vi "UI Array to KH Settings.vi"(4 "Bandwidth Filter":bool, 6 "DC Coupled":bool, 7 "KH Ch Ring":refnum<vi>, 8 "Default Shunt Resistor":T1=enum."50 Ohms", 9 "KH All Buttons":T15(ring), 10 "UI Channels []":T2[](array[typedef]) {"KH"."Channel" items=["A 1"]}, 11 "KH Ch Settings in":cluster{"Channel Setting":T10}[](array[cluster])) -> (2 "UI Channels [] out":T2[](array[typedef]) {"KH"."Channel" items=["A 1"]}, 3 "KH Ch Settings out":cluster{"Channel Setting":T10}[](array[cluster]))   [LabVIEW 2016, in "Control Experiment UI.lvclass"]
uses:
  Control Experiment UI.lvclass
  Typedefs/UI Channels--Cluster.ctl
  Typedefs/UI Channels.AI--Cluster.ctl
  Typedefs/UI Channels.Device--Cluster.ctl
  Control Experiment SM/Typedefs/KH Mode-enum.ctl
  Typedefs/UI Channels.KH--Cluster.ctl
  <userlib>/LevyLab/Krohn Hite 7008/typedefs/Input Configuration-Enum.ctl
  <userlib>/LevyLab/Krohn Hite 7008/typedefs/Gain-Enum.ctl
  <userlib>/LevyLab/Krohn Hite 7008/typedefs/Shunt-Enum.ctl
  Typedefs/UI Channels.AO--Cluster.ctl
  <userlib>/LevyLab/Krohn Hite 7008/typedefs/SetAll-Array.ctl
  <userlib>/LevyLab/Krohn Hite 7008/typedefs/SetAll-Cluster.ctl
  <userlib>/LevyLab/Krohn Hite 7008/typedefs/Channel-Enum.ctl
  <userlib>/LevyLab/Krohn Hite 7008/typedefs/Filter-Enum.ctl
  <userlib>/LevyLab/Krohn Hite 7008/typedefs/Coupling-Enum.ctl
  <userlib>/LevyLab/Krohn Hite 7008/Instrument.KH7008.lvclass
  Control Experiment SM/Control Experiment SM.lvclass
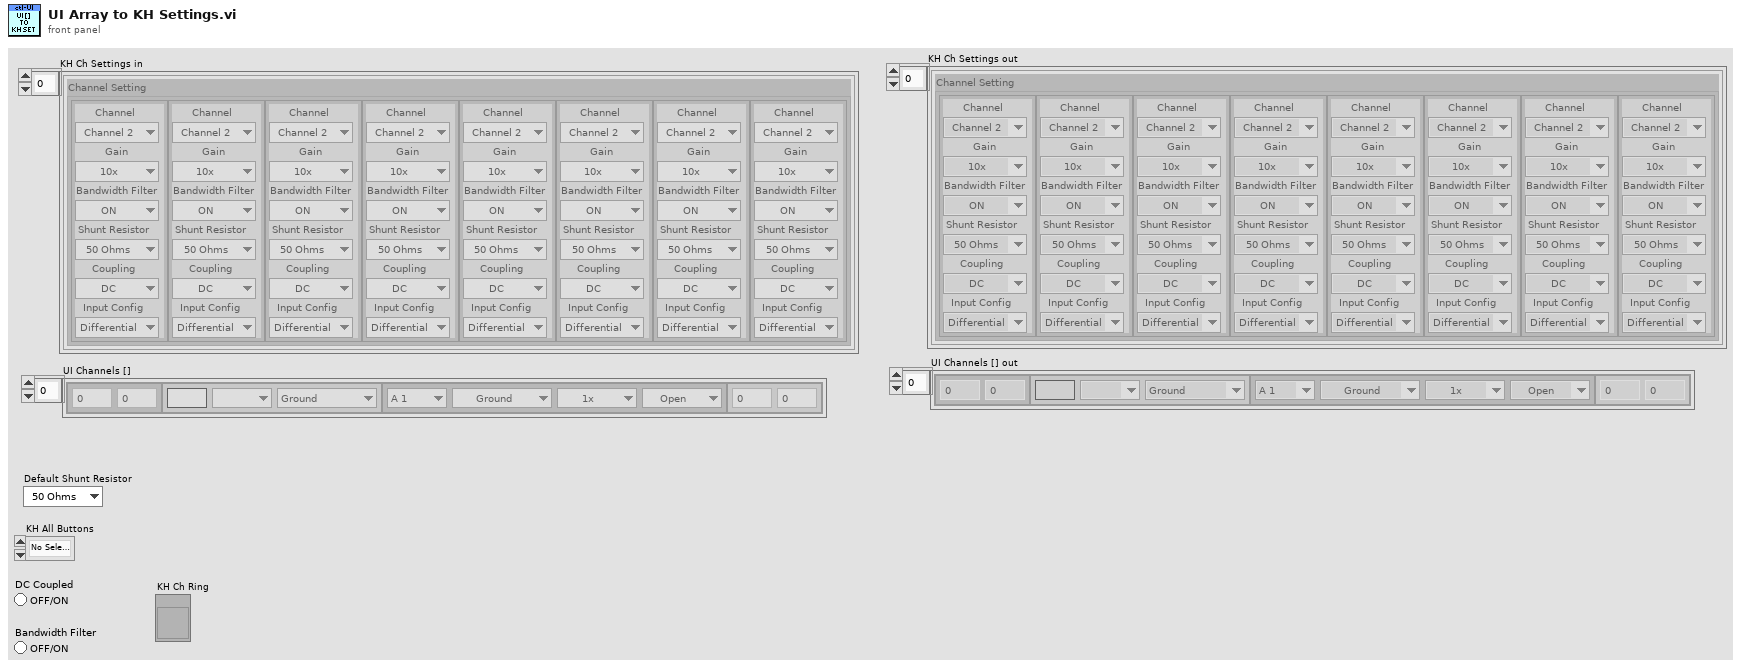
[diagram p1: front panel]
types:
  T1 = typedef "Instrument.KH7008.lvclass/Shunt-Enum.ctl" = enum16{"Open", "50 Ohms", "500 Ohms", "5k Ohms", "50k Ohms", "10M Ohm"}
  T2 = typedef "Control Experiment UI.lvclass/UI Channels--Cluster.ctl" = cluster{"AI":T3, "Device":T4, "KH":T6, "AO":T9}
  T3 = typedef "Control Experiment UI.lvclass/UI Channels.AI--Cluster.ctl" = cluster{"Channel":u32, "Gain":dbl}
  T4 = typedef "Control Experiment UI.lvclass/UI Channels.Device--Cluster.ctl" = cluster{"Electrode":string, "Configuration":T5, "Label":u16}
  T5 = typedef "Control Experiment SM.lvclass/KH Mode-enum.ctl" = enum16{"Ground", "Current", "Voltage (SE)", "Voltage (Diff)", "Gate"}
  T6 = typedef "Control Experiment UI.lvclass/UI Channels.KH--Cluster.ctl" = cluster{"Channel":u16, "Configuration":T7, "Gain":T8, "Shunt Resistor":T1}
  T7 = typedef "Instrument.KH7008.lvclass/Input Configuration-Enum.ctl" = enum16{"Ground", "SE+ (-gnd)", "SE- (+gnd)", "Differential"}
  T8 = typedef "Instrument.KH7008.lvclass/Gain-Enum.ctl" = enum16{"1x", "10x", "100x", "1000x"}
  T9 = typedef "Control Experiment UI.lvclass/UI Channels.AO--Cluster.ctl" = cluster{"Channel":u32, "Gain":dbl}
  T10 = typedef "Instrument.KH7008.lvclass/SetAll-Array.ctl" = T11[]
  T11 = typedef "Instrument.KH7008.lvclass/SetAll-Cluster.ctl" = cluster{"Channel":T12, "Gain":T8, "Bandwidth Filter":T13, "Shunt Resistor":T1, "Coupling":T14, "Input Config":T7}
  T12 = typedef "Instrument.KH7008.lvclass/Channel-Enum.ctl" = enum16{"Channel 1", "Channel 2", "Channel 3", "Channel 4", "Channel 5", "Channel 6", "Channel 7", "Channel 8"}
  T13 = typedef "Instrument.KH7008.lvclass/Filter-Enum.ctl" = enum16{"OFF", "ON"}
  T14 = typedef "Instrument.KH7008.lvclass/Coupling-Enum.ctl" = enum16{"AC", "DC"}
  T15 = enum32{"No Selection", "All Ground", "All Differential"}
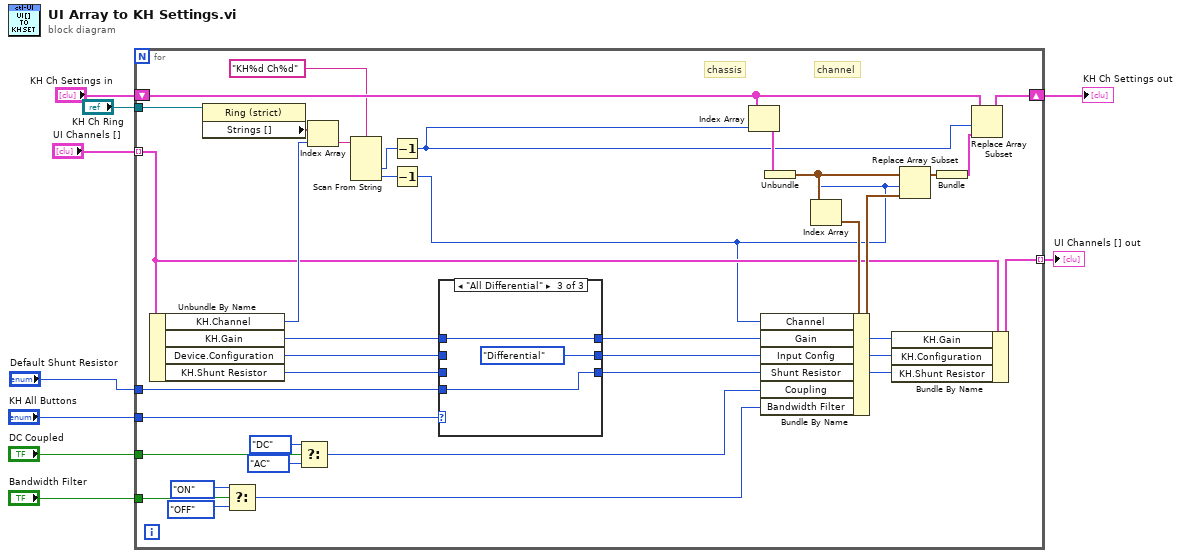
[diagram p0: block diagram]
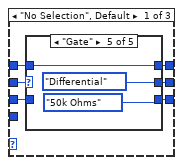
[diagram p2: hidden frame]
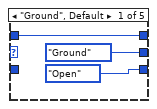
[diagram p3: hidden frame]
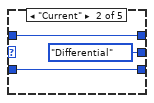
[diagram p4: hidden frame]
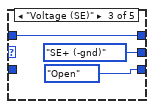
[diagram p5: hidden frame]
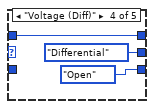
[diagram p6: hidden frame]
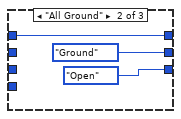
[diagram p7: hidden frame]
diagram:
  n1 = for {
    tunnel: "UI Channels []" -> [w21] mode=indexing
    shift-right: [w42] -> w5
    shift-left: "KH Ch Settings in" -> [w41]
    tunnel: "Bandwidth Filter" -> [w32]
    tunnel: "DC Coupled" -> [w28]
    tunnel: [w22] -> w8 mode=indexing
    tunnel: "KH All Buttons" -> [w15]
    tunnel: "KH Ch Ring" -> [w26]
    tunnel: "Default Shunt Resistor" -> [w10]
    # "channel"
    # "chassis"
    n2 = Unbundle By Name(w21) -> ("KH.Channel"=w37:u16, "KH.Gain"=w17:T8, "Device.Configuration"=w14:T5, "KH.Shunt Resistor"=w13:T1)
    n3 = property on="Property Node" class="Ring (strict)"(reference=w26) -> ("Strings []"=w38:string[])  [unwired: 1 in, 2 out]
    n4 = Select(t=Filter-Enum."ON" ("Bandwidth Filter"), s=w32, f=Filter-Enum."OFF" ("Bandwidth Filter")) -> (s? t:f=w19:T13)
    n5 = Select(t=Coupling-Enum."DC" ("Coupling"), s=w28, f=Coupling-Enum."AC" ("Coupling")) -> (s? t:f=w27:T14)
    n6 = Index Array(array=w38, index=w37) -> (element=w36:string)
    n7 = Scan From String(format string="KH%d Ch%d", input string=w36) -> (output 1=w35:i32, output 2=w34:i32)  [unwired: 4 in, 3 out]
    n8 = Decrement(x=w35) -> (x-1=w25:i32)
    n9 = Decrement(x=w34) -> (x-1=w18:i32)
    n10 = case shown="\"All Differential\"" w15 {
      tunnel: w14 -> [w46 _ _]
      tunnel: [w50 Input_Configuration-Enum."Ground" ("Input Config") Input_Configuration-Enum."Differential" ("Input Config")] -> w12
      tunnel: w17 -> [w49 w68 w71]
      tunnel: [w48 w68 w71] -> w16
      tunnel: [w47 Shunt-Enum."Open" ("Shunt Resistor") w69] -> w11
      tunnel: w13 -> [w45 _ _]
      tunnel: w10 -> [_ _ w69]
      frame "No Selection", Default {
        n11 = case shown="\"Gate\"" w46 {
          tunnel: [Input_Configuration-Enum."Ground" ("Input Config") Input_Configuration-Enum."Differential" ("Input Config") Input_Configuration-Enum."SE+ (-gnd)" ("Input Config") Input_Configuration-Enum."Differential" ("Input Config") Input_Configuration-Enum."Differential" ("Input Config")] -> w50
          tunnel: [Shunt-Enum."Open" ("Shunt Resistor") w54 Shunt-Enum."Open" ("Shunt Resistor") Shunt-Enum."Open" ("Shunt Resistor") Shunt-Enum."50k Ohms" ("Shunt Resistor")] -> w47
          tunnel: w49 -> [w51 w55 w58 w62 w64]
          tunnel: [w51 w55 w58 w62 w64] -> w48
          tunnel: w45 -> [_ w54 _ _ _]
          frame "Ground", Default {
          }
          frame "Current" {
          }
          frame "Voltage (SE)" {
          }
          frame "Voltage (Diff)" {
          }
          frame "Gate" {
          }
        }
      }
      frame "All Ground" {
      }
      frame "All Differential" {
      }
    }
    n12 = Index Array(array=w41, index=w25) -> (element=w43:cluster{"Channel Setting":T10})
    n13 = Unbundle(w43) -> ("Channel Setting"=w20:T10)
    n14 = Index Array(array=w20, index=w18) -> (element=w40:T11)
    n15 = Bundle By Name(cluster=w40, "Channel"=w18, "Gain"=w16, "Input Config"=w12, "Shunt Resistor"=w11, "Coupling"=w27, "Bandwidth Filter"=w19) -> (w24:T11)
    n16 = Bundle By Name(cluster=w21, "KH.Gain"=w16, "KH.Configuration"=w12, "KH.Shunt Resistor"=w11) -> (w22:T2)
    n17 = Replace Array Subset(array=w20, new element=w24, index=w18) -> (w44:T10)
    n18 = Bundle("Channel Setting"=w44) -> (w23:cluster{"Channel Setting":T10})  [unwired: 1 in]
    n19 = Replace Array Subset(array=w41, new element=w23, index=w25) -> (w42:cluster{"Channel Setting":T10}[])
  }
  "UI Channels [] out" <- w8
  "KH Ch Settings out" <- w5
